vi "waitx2.vi"(2 "timeoutms":u32=120000, 3 "String Value 2":string(combo)="pending", 4 "String Value":string(combo)="stoped", 5 "连接ID":refnum<k5>) -> (0 "字符串":string, 1 "连接ID 2":refnum<k5>)   [LabVIEW 2017]
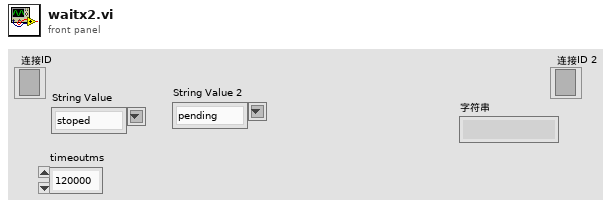
[diagram p1: front panel]
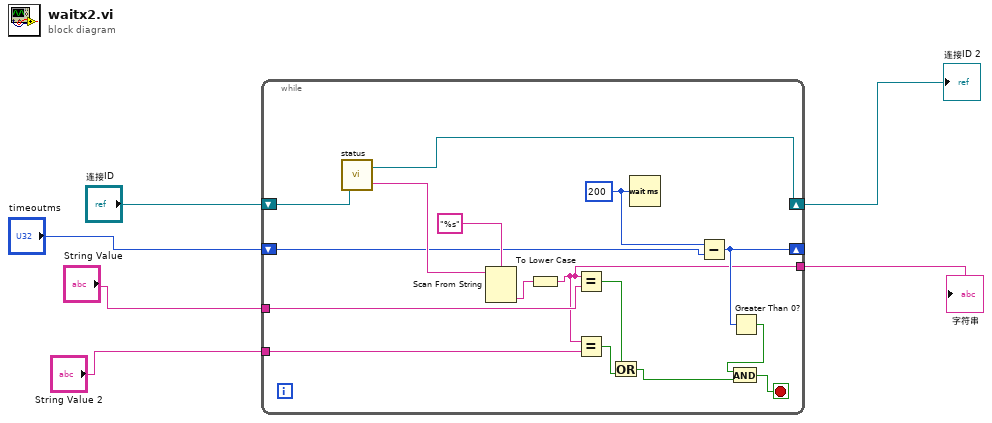
[diagram p0: block diagram]
diagram:
  n1 = while {
    shift-right: [w21] -> w3
    shift-left: "连接ID" -> [w22]
    shift-right: [w15] -> _
    shift-left: "timeoutms" -> [w16]
    tunnel: "String Value" -> [w12]
    tunnel: "String Value 2" -> [w11]
    tunnel: [w7] -> w1
    stop <- w13 stop-if-true
    w17 = u32 200 ("等待时间（毫秒）")
    n2 = call "status.vi"("连接ID"=w22) -> ("连接ID输出"=w21:refnum<k5>, "String Value"=w20:string)
    n3 = Scan From String(format string="%s" ("格式字符串"), input string=w20) -> (output 1=w18:string)  [unwired: 3 in, 3 out]
    n4 = To Lower Case(string=w18) -> (all lower case string=w7:string)
    n5 = Equal?(x=w7, y=w12) -> (x = y?=w9:bool)
    n6 = Equal?(x=w7, y=w11) -> (x = y?=w10:bool)
    n7 = Or(x=w9, y=w10) -> (x .or. y?=w8:bool)
    n8 = Wait (ms)(milliseconds to wait=w17) -> ()  [unwired: 1 out]
    n9 = Subtract(x=w17, y=w16) -> (x-y=w15:u32)
    n10 = Greater Than 0?(x=w15) -> (x > 0?=w14:bool)
    n11 = And(x=w14, y=w8) -> (x .and. y?=w13:bool)
  }
  "连接ID 2" <- w3
  "字符串" <- w1
